vi "Error Query.vi"(8 "error in (no error)":errorcluster, 11 "VISA resource name":refnum<visa-resource-name>) -> (0 "error out":errorcluster, 1 "Error Message":string, 2 "Error Code":i32[](array[numeric]), 3 "VISA resource name out":refnum<visa-resource-name>)   [LabVIEW 2020, in "GPP.lvlib"]
uses:
  GPP.lvlib
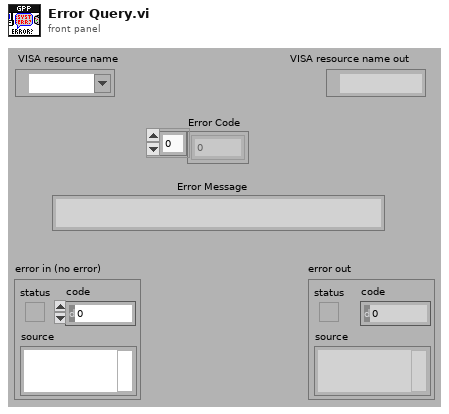
[diagram p1: front panel]
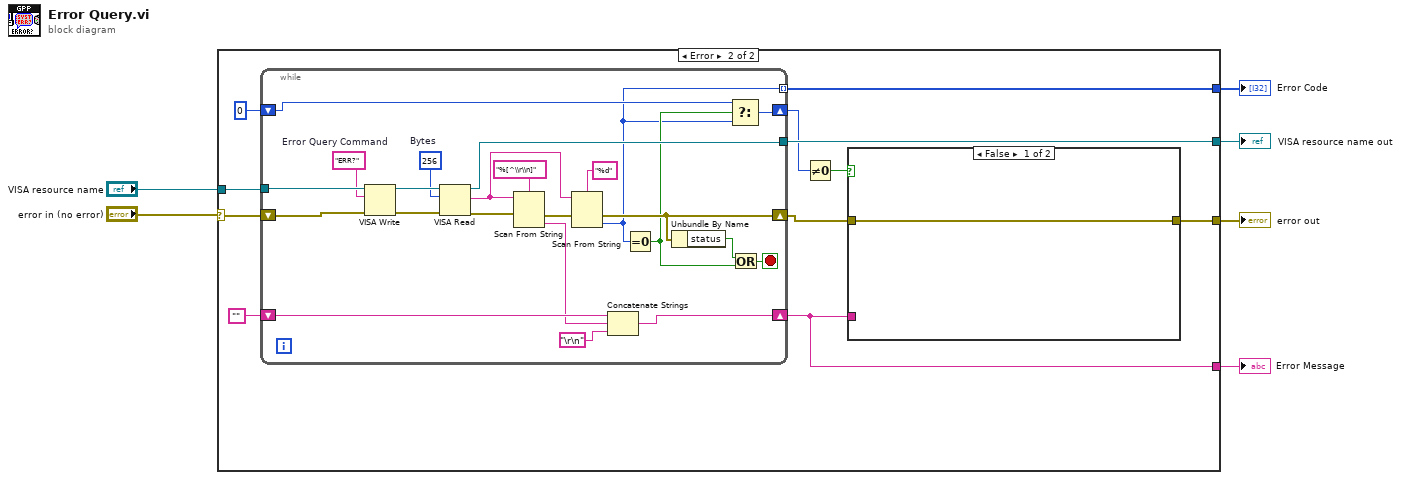
[diagram p0: block diagram]
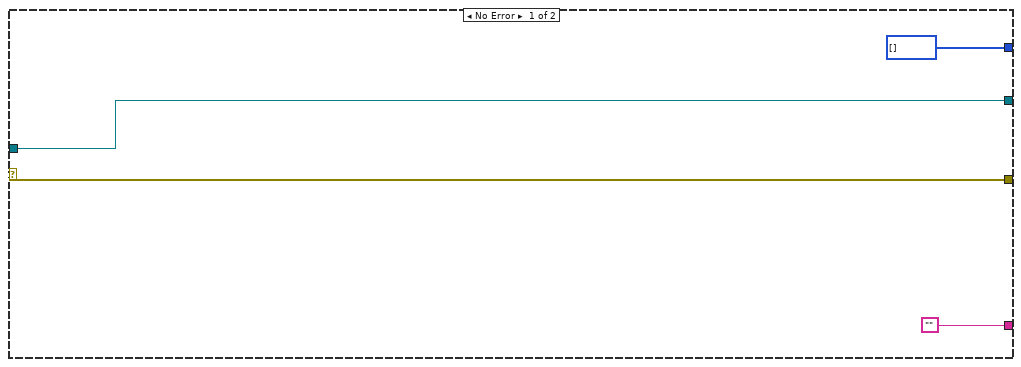
[diagram p2: hidden frame]
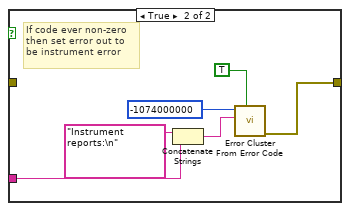
[diagram p3: hidden frame]
diagram:
  n1 = case shown="Error" "error in (no error)" {
    selector: "error in (no error)" -> [w7 w13]
    tunnel: [w10 w21] -> w6
    tunnel: "VISA resource name" -> [w10 w12]
    tunnel: [w7 w14] -> w5
    tunnel: ["" ("Empty String Constant") w15] -> w4
    tunnel: [i32[] [] w17] -> w3
    frame No Error {
    }
    frame Error {
      n2 = while {
        tunnel: [w51] -> w21
        tunnel: w12 -> [w50]
        shift-right: [w38] -> w15
        shift-left: "" ("Empty String Constant") -> [w41]
        shift-right: [w36] -> w18
        shift-left: 0 -> [w37]
        shift-right: [w34] -> w11
        shift-left: w13 -> [w35]
        tunnel: [w29] -> w17 mode=indexing
        stop <- w44 stop-if-true
        w48 = u32 256  # Bytes
        w46 = "ERR?"  # Error Query Command
        n3 = VISA Write(VISA resource name=w50, write buffer=w46, error in (no error)=w35) -> (VISA resource name out=w49:refnum<visa-resource-name>, error out=w47:errorcluster)  [unwired: 1 out]
        n4 = VISA Read(VISA resource name=w49, byte count=w48, error in (no error)=w47) -> (VISA resource name out=w51:refnum<visa-resource-name>, read buffer=w42:string, error out=w33:errorcluster)  [unwired: 1 out]
        n5 = Scan From String(format string="%[^\\r\\n]", input string=w42, error in=w33) -> (error out=w32:errorcluster, output 1=w39:string)  [unwired: 1 in, 3 out]
        n6 = Scan From String(format string="%d", input string=w42, error in=w32) -> (error out=w34:errorcluster, output 1=w29:i32)  [unwired: 1 in, 3 out]
        n7 = Concatenate Strings(w41, w39, "\r\n" ("End of Line Constant")) -> (w38:string)
        n8 = Equal To 0?(x=w29) -> (x = 0?=w30:bool)
        n9 = Unbundle By Name(w34) -> ("status"=w31:bool)
        n10 = Select(t=w37, s=w30, f=w29) -> (s? t:f=w36:i32)
        n11 = Or(x=w31, y=w30) -> (x .or. y?=w44:bool)
      }
      n12 = Not Equal To 0?(x=w18) -> (x != 0?=w16:bool)
      n13 = case shown="False" w16 {
        tunnel: w15 -> [_ w27]
        tunnel: [w22 w23] -> w14
        tunnel: w11 -> [w22 _]
        frame False {
        }
        frame True {
          # "If code ever non-zero\nthen set error out to\nbe instrument error"
          n14 = Concatenate Strings("Instrument reports:\n" ("Source"), w27) -> (w24:string)
          n15 = call <vilib>:"Error Cluster From Error Code.vi"("show call chain? (False)"=TRUE, "error message (\"\")"=w24, "error code (0)"=-1074000000 ("Code")) -> ("error out"=w23:errorcluster)  [unwired: 1 in, 5 out]
        }
      }
    }
  }
  "VISA resource name out" <- w6
  "error out" <- w5
  "Error Message" <- w4
  "Error Code" <- w3
